vi "PDSS - Turn Trigger Light On.vi"(8 "error in (no error)":errorcluster) -> (0 "error out":errorcluster, 3 "Trigger Started":bool)   [LabVIEW 2014]
doc: "Use this template to build a VI to use as a subVI."
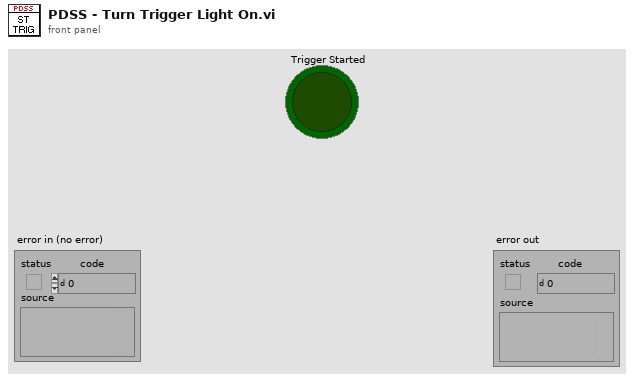
[diagram p1: front panel]
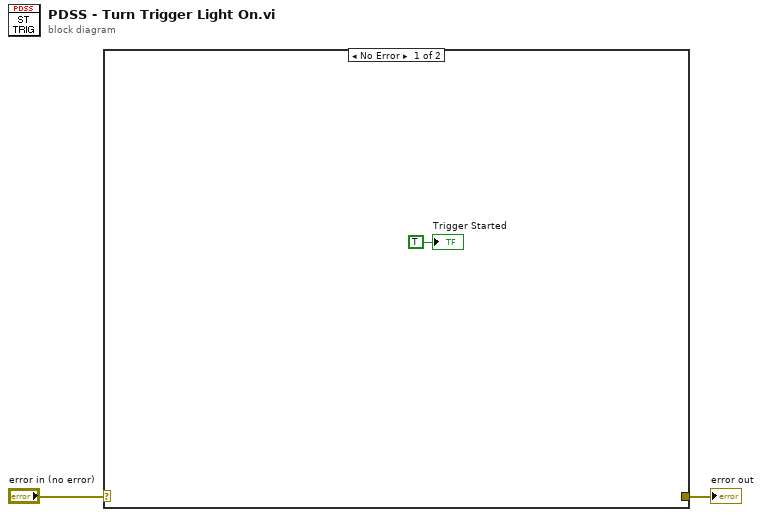
[diagram p0: block diagram]
diagram:
  n1 = case shown="No Error" "error in (no error)" {
    selector: "error in (no error)" -> [_ w4]
    tunnel: [_ w4] -> w1
    frame No Error {
      "Trigger Started" <- TRUE ("Trigger Started")
    }
    frame Error {
    }
  }
  "error out" <- w1
